vi "(SubVI)_Control_Save_Dpp_bin.vi"(9 "Frm#":dbl=1310.0, 10 "Dpp_bsln":dbl=1.5694465244142645e-05, 11 "refnum in":refnum<file>) -> (0 "error out":errorcluster, 3 "refnum out":refnum<file>)   [LabVIEW 2019]
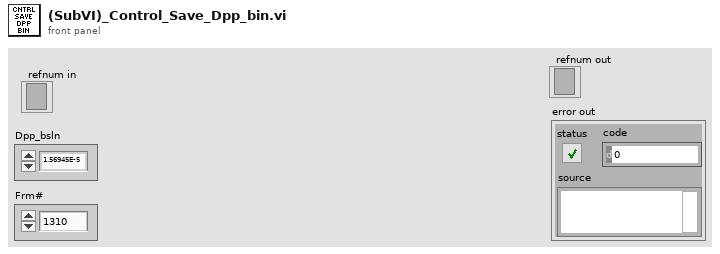
[diagram p1: front panel]
types:
  T1 = enum16{"big-endian, network order", "native, host order", "little-endian"}
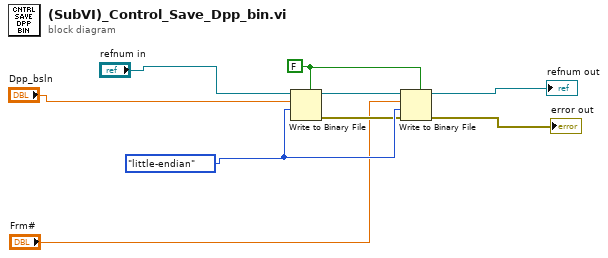
[diagram p0: block diagram]
diagram:
  w7 = T1."little-endian" ("byte order (0:big-endian, network order)")
  w9 = FALSE ("prepend array or string size? (T)")
  n1 = Write to Binary File(file (use dialog)="refnum in", data="Dpp_bsln", 5:w9, 9:w7) -> (refnum out=w8:refnum<file>, error out=w6:errorcluster)  [unwired: 2 in, 1 out]
  n2 = Write to Binary File(file (use dialog)=w8, data="Frm#", error in=w6, 5:w9, 9:w7) -> (refnum out=→"refnum out":refnum<file>, error out=→"error out":errorcluster)  [unwired: 1 in, 1 out]
